vi "Take_Data_on_the_Move.vi"(3 "Mode":T5, 5 "Traverse line In":T2 {"Row Duration (mins)" format="%#.1f"; "Row No" min=0; "Trace Gas Concentration (%)" min=0.0 format="%#.2f"; "Emission Rate (l/min)" format="%#.2f"; "Tunnel Speed" format="%#.2f"; "Start X" format="%#.2f"; "Start Y" format="%#.2f"; "Start Z" format="%#.2f"; "End X" format="%#.2f"; "End Y" format="%#.2f"; "End Z" format="%#.2f"; "Averaging time (min)" min=0.0 format="%#.2f"}) -> (0 "Error Message":string, 1 "Status":T1, 2 "Traverse line Out":T2 {"Row Duration (mins)" format="%#.1f"; "Row No" min=0; "Trace Gas Concentration (%)" min=0.0 format="%#.2f"; "Emission Rate (l/min)" format="%#.2f"; "Tunnel Speed" format="%#.2f"; "Start X" format="%#.2f"; "Start Y" format="%#.2f"; "Start Z" format="%#.2f"; "End X" format="%#.2f"; "End Y" format="%#.2f"; "End Z" format="%#.2f"; "Averaging time (min)" min=0.0 format="%#.2f"})   [LabVIEW 2010]
uses:
  Gen Trav/Multi_Run_Status.ctl
  Globals/Dynamic_call_global.ph.vi
  Controls/Save_Data.ctl
  Controls/Setup.ctl
  Gen Trav/Spacing.ctl
  Gen Trav/Traverse_cluster.ctl
  Controls/User_Specific_mode.ctl
  Controls/Multi_run_mode.ctl
panel:
  # "X           Y            Z"
  # "Start"
  # "End"
  # "X           Y            Z"
  # "Start"
  # "End"
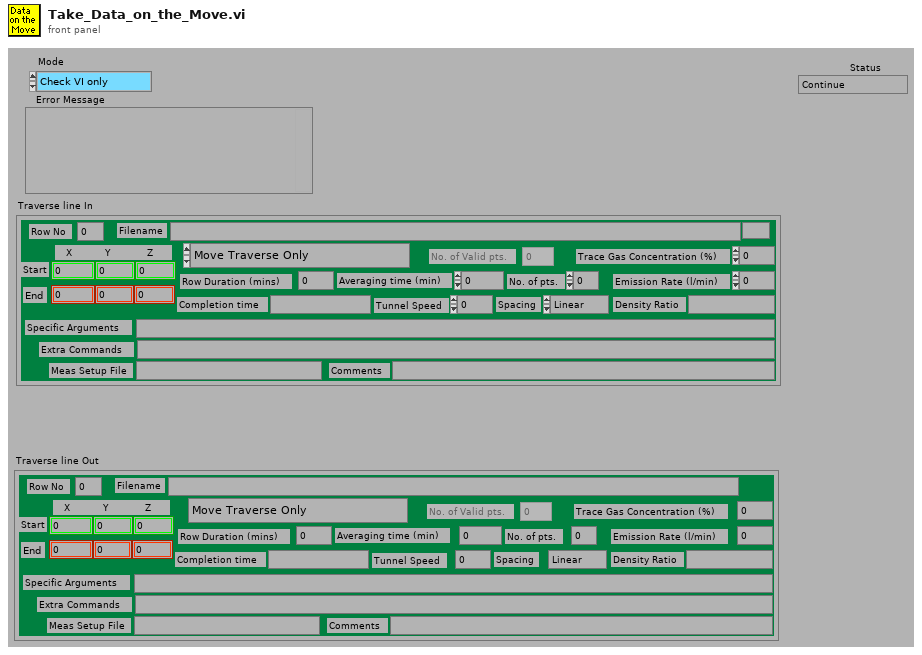
[diagram p1: front panel]
types:
  T1 = typedef "Multi_Run_Status.ctl" = enum16{"Continue", "Jump to Next Point", "Jump to Next Row", "Jump To Fall Back", "Terminate Run"}
  T2 = typedef "Traverse_cluster.ctl" = cluster{"Start X":dbl, "Start Y":dbl, "Start Z":dbl, "End X":dbl, "End Y":dbl, "End Z":dbl, "No. of pts.":i32, "Spacing":T3, "Filename":path, "Tunnel Speed":dbl, "Averaging time (min)":dbl, "Extra Commands":string, "Specific Arguments":string, "Emission Rate (l/min)":dbl, "Trace Gas Concentration (%)":dbl, "Density Ratio":string, "Comments":string, "Row No":i32, "Row Type Selector":T4, "Completion time":string, "Row Duration (mins)":dbl, "No. of Valid pts.":i32, "Meas Setup File":string}
  T3 = typedef "Spacing.ctl" = enum16{"Linear", "Log", "Gauss", "Specified", "N/A"}
  T4 = typedef "Multi_run_mode.ctl" = enum16{"Move Traverse Only", "Set Tunnel Speed Only", "Set Source Only", "Set Measurement Conditions", "Single Measurement", "Vertical Profile", "Lateral Profile", "Longitudinal Profile", "Explore Volume", "Multi-Axis Profile", "Auto Calibrate", "Meas Fast FID Bkgnd", "Check Beam Power", "Scanning Valve Measurement", "Run VI Named:", "Set ADAM Ch", "Wait (minutes)", "Send Message", "Synchronize With:", "Fall Back to this Row", "Turn Off Row Repeating", "Blank Row"}
  T5 = typedef "User_Specific_mode.ctl" = enum16{"Check VI only", "Run VI"}
  T6 = typedef "Setup.ctl" = enum16{"Run Program", "Show Setup", "Save Current Setup", "Setup Front Panel"}
  T7 = typedef "Save_Data.ctl" = enum16{"Save No Data", "Save Data"}
  T8 = typedef "Status_Cluster.ctl" = cluster{"Status":T1, "Error Type":string, "Error Description":string}
  T9 = typedef "Rendezvous RefNum" = refnum<k1>
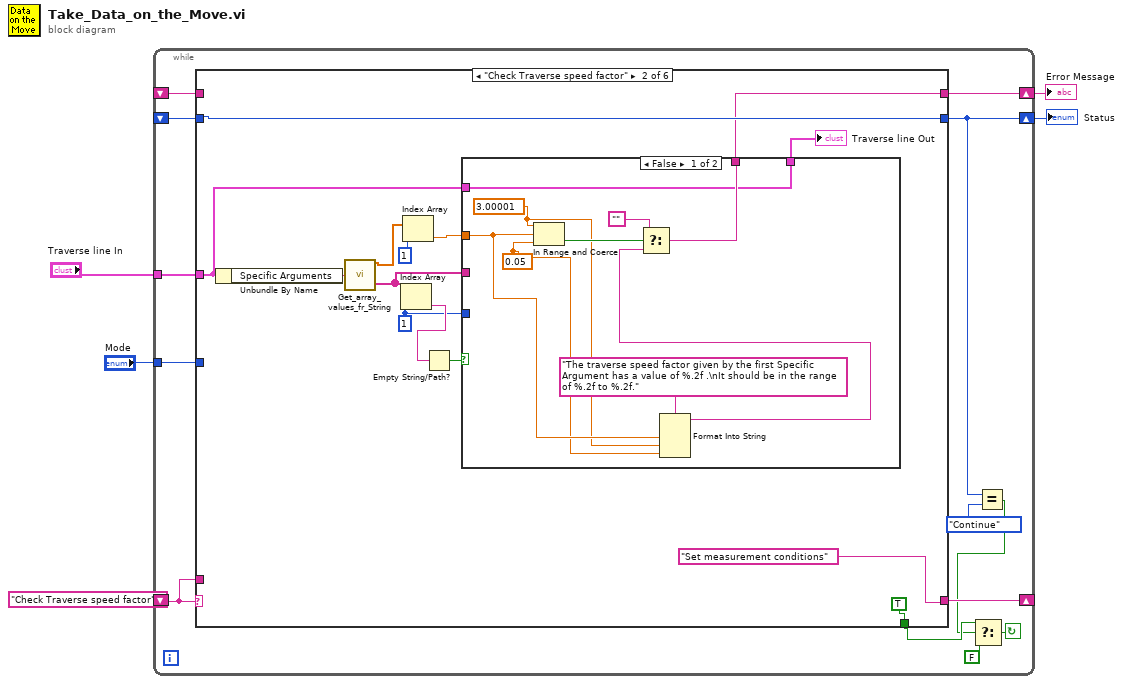
[diagram p0: block diagram]
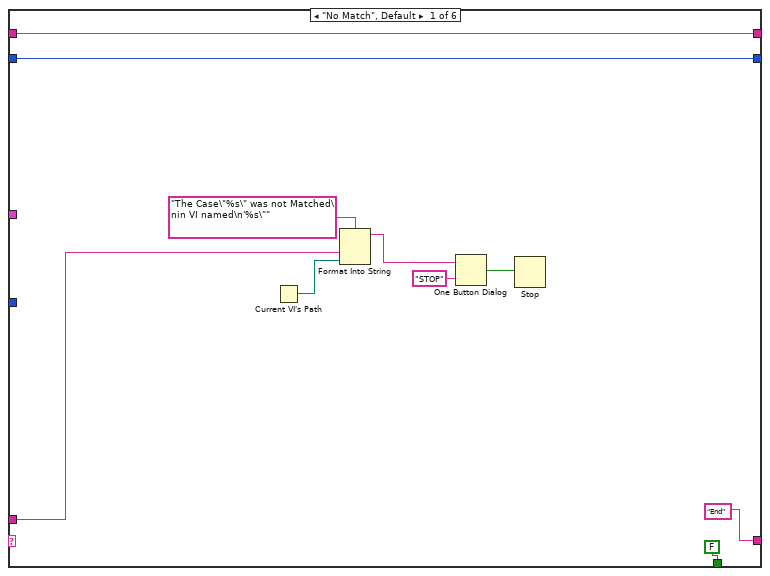
[diagram p2: hidden frame]
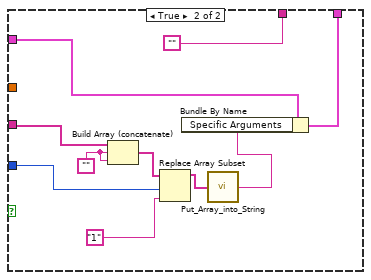
[diagram p3: hidden frame]
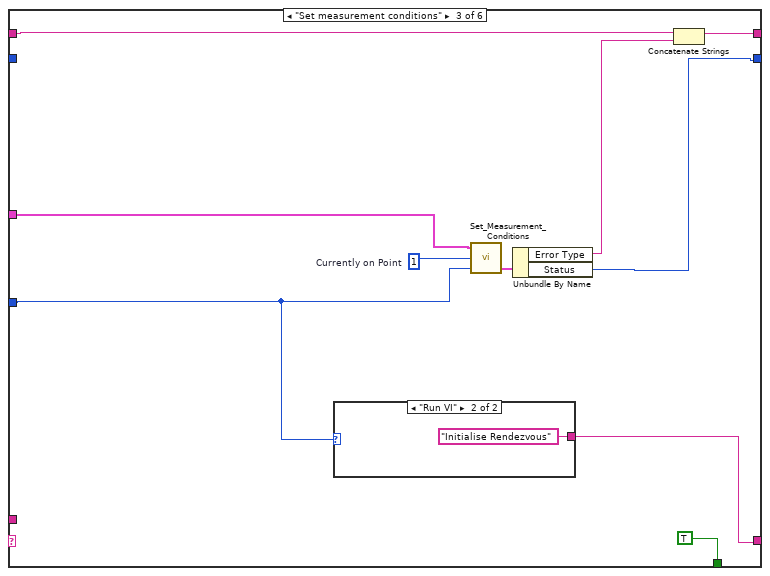
[diagram p4: hidden frame]
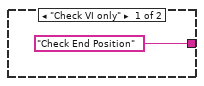
[diagram p5: hidden frame]
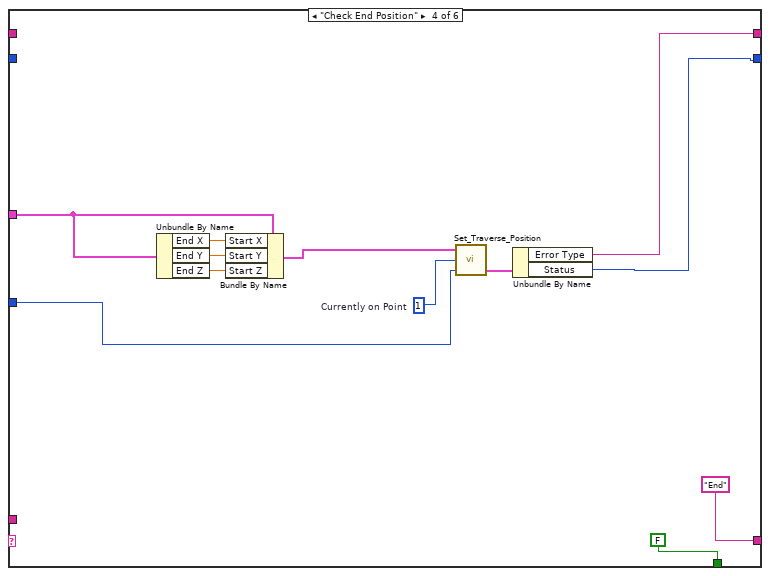
[diagram p6: hidden frame]
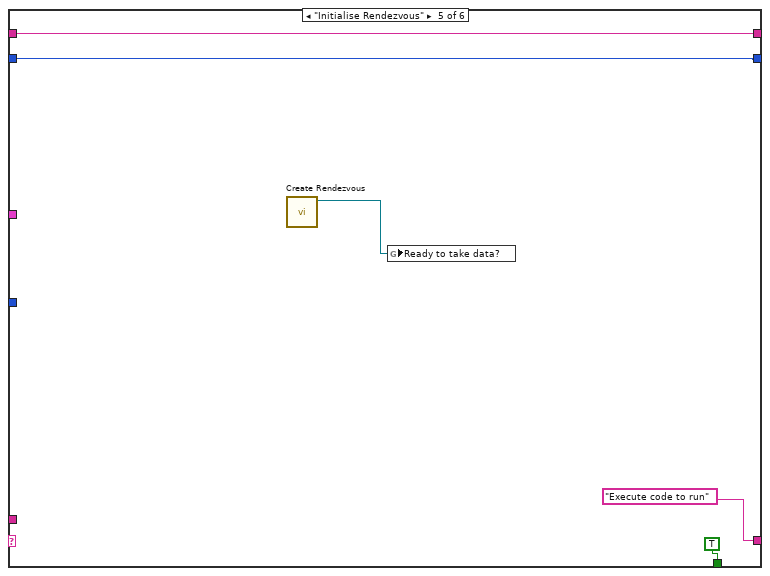
[diagram p7: hidden frame]
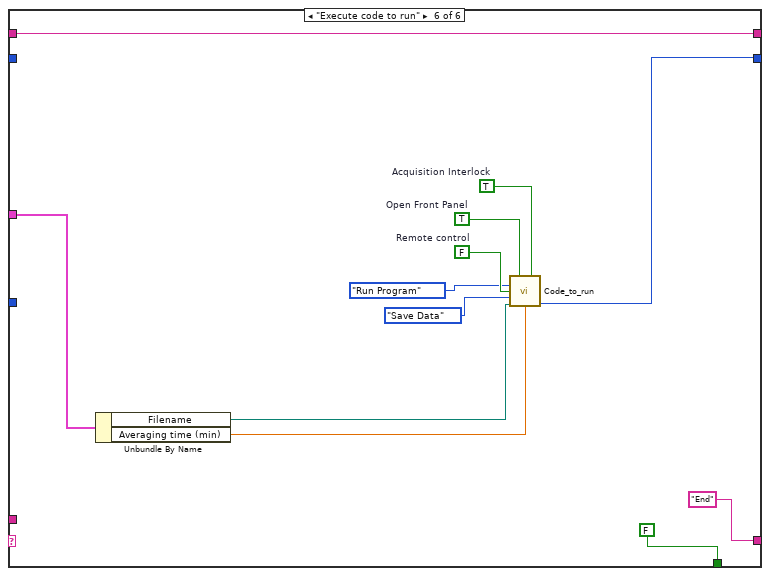
[diagram p8: hidden frame]
diagram:
  n1 = while {
    shift-left: _ -> [w13]
    shift-right: [w8] -> w2
    shift-left: _ -> [w16]
    shift-right: [w14] -> w3
    tunnel: "Traverse line In" -> [w17]
    tunnel: "Mode" -> [w18]
    shift-left: "Check Traverse speed factor" -> [w15]
    shift-right: [w12] -> _
    stop <- w6 continue-if-true
    n2 = case shown="\"Check Traverse speed factor\"" w15 {
      tunnel: w17 -> [_ w35 w67 w85 _ w95]
      tunnel: w18 -> [_ _ w68 w77 _ _]
      tunnel: [FALSE ("Update Datum Powers?") TRUE ("Update Datum Powers?") TRUE ("Update Datum Powers?") FALSE ("Update Datum Powers?") TRUE ("Update Datum Powers?") FALSE ("Update Datum Powers?")] -> w11
      tunnel: ["End" "Set measurement conditions" w63 "End" "Execute code to run" "End"] -> w12
      tunnel: w16 -> [w23 _ w65 _ w87 w94]
      tunnel: [w23 w29 w64 w74 w87 w94] -> w14
      tunnel: w15 -> [w20 _ _ _ _ _]
      tunnel: w13 -> [w19 w38 _ _ w86 _]
      tunnel: [w19 w38 w69 w83 w86 w98] -> w8
      frame "No Match", Default {
        n3 = Current VI's Path() -> (path=w24:path)
        n4 = Format Into String(format string="The Case\"%s\" was not Matched\nin VI named\n'%s\"" ("Format String"), w20, w24) -> (resulting string=w27:string)  [unwired: 2 in, 1 out]
        n5 = One Button Dialog(message=w27, button name ("OK")="STOP") -> (true=w25:bool)
        n6 = Stop(stop? (T)=w25) -> ()
      }
      frame "Check Traverse speed factor" {
        w32 = 1 ("index")
        n7 = Unbundle By Name(w35) -> ("Specific Arguments"=w42:string)
        n8 = call "Get_array_values_fr_String.vi"("String Value"=w42) -> ("Numeric Array"=w41:dbl[], "String array"=w31:string[])
        n9 = Index Array(array=w31, index=w32) -> (element=w34:string)
        n10 = Index Array(array=w41, index=1) -> (element=w39:dbl)
        n11 = Empty String/Path?(string/path=w34) -> (empty?=w33:bool)
        n12 = case shown="False" w33 {
          tunnel: w39 -> [w49 _]
          tunnel: [w44 ""] -> w29
          tunnel: [w43 w55] -> w36
          tunnel: w35 -> [w43 w56]
          tunnel: w32 -> [_ w59]
          tunnel: w31 -> [_ w54]
          frame False {
            w47 = 0.05 ("lower limit")
            w48 = 3.00001 ("upper limit")
            n13 = In Range and Coerce(upper limit=w48, x=w49, lower limit=w47) -> (In Range?=w51:bool)  [unwired: 1 out]
            n14 = Format Into String(format string="The traverse speed factor given by the first Specific Argument has a value of %.2f .\nIt should be in the range of %.2f to %.2f.", w49, w48, w47) -> (resulting string=w45:string)  [unwired: 2 in, 1 out]
            n15 = Select(t="", s=w51, f=w45) -> (s? t:f=w44:string)
          }
          frame True {
            w53 = ""
            n16 = Build Array (concatenate)(w54, w53, w53) -> (w52:string[])
            n17 = Replace Array Subset(array=w52, new element="1" ("new element/subarray"), index=w59) -> (w60:string[])
            n18 = call "Put_Array_into_String.vi"("String array"=w60) -> ("String Value"=w57:string)
            n19 = Bundle By Name(cluster=w56, "Specific Arguments"=w57) -> (w55:T2)
          }
        }
        "Traverse line Out" <- w36
      }
      frame "Set measurement conditions" {
        w71 = 1  # Currently on Point
        n20 = case shown="\"Run VI\"" w68 {
          tunnel: ["Check End Position" "Initialise Rendezvous"] -> w63
          frame "Check VI only" {
          }
          frame "Run VI" {
          }
        }
        n21 = call "Set_Measurement_Conditions.vi"("Simulate/Run"=w68, "Currently on Point"=w71, "Traverse line"=w67) -> ("Status Cluster"=w70:T8)  [unwired: 2 out]
        n22 = Unbundle By Name(w70) -> ("Error Type"=w66:string, "Status"=w69:T1)
        n23 = Concatenate Strings(w65, w66) -> (w64:string)
      }
      frame "Check End Position" {
        w78 = 1  # Currently on Point
        n24 = Unbundle By Name(w85) -> ("End X"=w82:dbl, "End Y"=w81:dbl, "End Z"=w80:dbl)
        n25 = Bundle By Name(cluster=w85, "Start X"=w82, "Start Y"=w81, "Start Z"=w80) -> (w76:T2)
        n26 = call "Set_Traverse_Position.vi"("Simulate/Run"=w77, "Currently on Point"=w78, "Traverse line"=w76) -> ("Status Cluster"=w75:T8)  [unwired: 2 out]
        n27 = Unbundle By Name(w75) -> ("Error Type"=w74:string, "Status"=w83:T1)
      }
      frame "Initialise Rendezvous" {
        n28 = call <vilib>:"Create Rendezvous.vi"() -> ("rendezvous"=w90:T9)  [unwired: 2 in, 5 out]
        n29 = global write "Dynamic_call_global.ph.vi" "Ready to take data?"(w90) -> ()
      }
      frame "Execute code to run" {
        w99 = TRUE  # Acquisition Interlock
        w100 = TRUE  # Open Front Panel
        w102 = FALSE  # Remote control
        n30 = Unbundle By Name(w95) -> ("Filename"=w91:path, "Averaging time (min)"=w101:dbl)
        n31 = call "Code_to_run.vi"("Open Front Panel"=w100, "Acquisition Interlock"=w99, "setup"=Setup."Run Program", "Remote control"=w102, "File"=Save_Data."Save Data", "Results Filename"=w91, "Averaging time (min)"=w101) -> ("Status"=w98:T1)  [unwired: 4 in, 4 out]
      }
    }
    n32 = Equal?(x=w8, y=Multi_Run_Status."Continue" ("Status")) -> (x = y?=w10:bool)
    n33 = Select(t=w11, s=w10, f=FALSE) -> (s? t:f=w6:bool)
  }
  "Status" <- w2
  "Error Message" <- w3
